vi "subvi.vi"(11 "Numeric 4":dbl) -> ()   [LabVIEW 2018]
panel:
  in  "Numeric 3":dbl
  out "Numeric 2":dbl
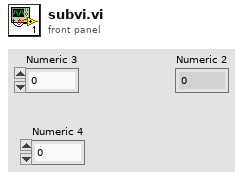
[diagram p1: front panel]
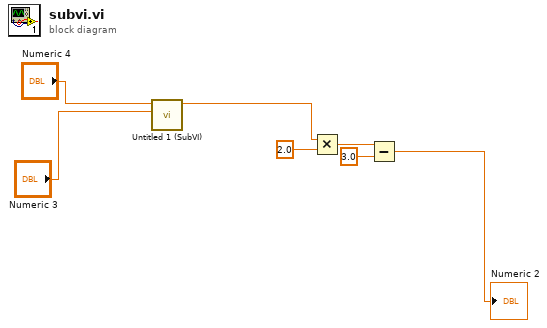
[diagram p0: block diagram]
diagram:
  n1 = call "Untitled 1 (SubVI).vi"("Numeric 3"="Numeric 3", "Numeric 4"="Numeric 4") -> ("Numeric"=w6:dbl)  [unwired: 9 in]
  n2 = Multiply(x=w6, y=2.0) -> (x*y=w4:dbl)
  n3 = Subtract(x=w4, y=3.0) -> (x-y=→"Numeric 2":dbl)
